vi "Model - Init.vi"(8 "error in (no error)":errorcluster) -> (0 "error out":errorcluster, 3 "View Model":T1)   [LabVIEW 2017]
doc: "Initialize all View Model Components."
uses:
  Controls/View Model.ctl
  Controls/Shared Model.ctl
  Error Handler/Controls/Error Model.ctl
  Error Handler/Controls/Error Data.ctl
  Error Handler/Controls/Error Type.ctl
  Error Handler/Controls/Error Source.ctl
  Configuration/Controls/Config Model.ctl
  Configuration/Controls/Config CMD.ctl
  Configuration/Controls/Config Command.ctl
  Controller/Controls/Controller Model.ctl
  Controller/Controls/Controller Overhead.ctl
  Controller/Controls/Controller Transaction.ctl
  Controller/Controls/Controller State.ctl
  Configuration/Controls/Config Data Record.ctl
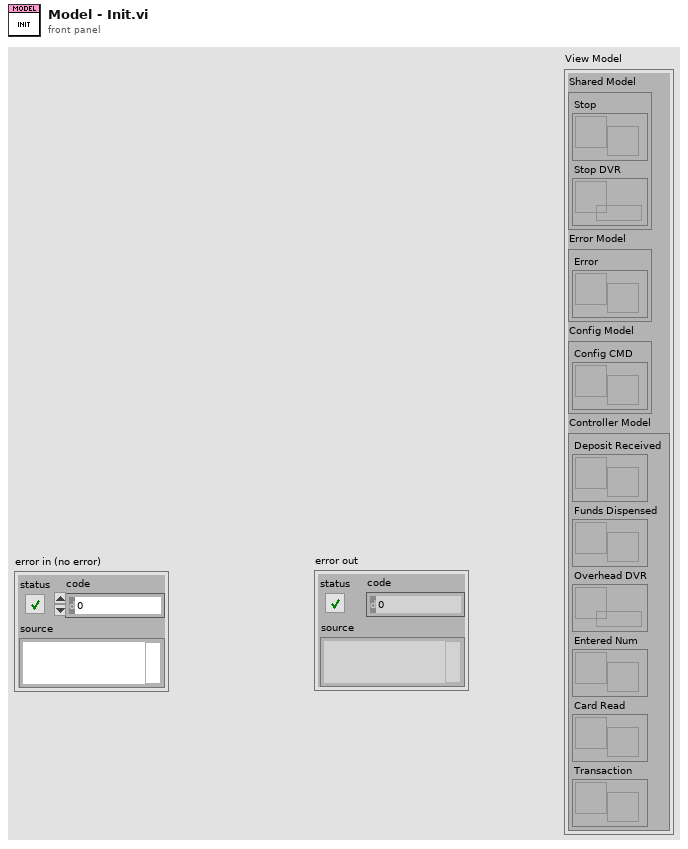
[diagram p1: front panel]
types:
  T1 = typedef "View Model.ctl" = cluster{"Shared Model":T2, "Error Model":T3, "Config Model":T4, "Controller Model":T5}
  T2 = typedef "Shared Model.ctl" = cluster{"Stop":refnum<user-event>, "Stop DVR":refnum<data-value>}
  T3 = typedef "Error Model.ctl" = cluster{"Error":refnum<user-event>}
  T4 = typedef "Config Model.ctl" = cluster{"Config CMD":refnum<user-event>}
  T5 = typedef "Controller Model.ctl" = cluster{"Deposit Received":refnum<user-event>, "Funds Dispensed":refnum<user-event>, "Overhead DVR":refnum<data-value>, "Entered Num":refnum<user-event>, "Card Read":refnum<user-event>, "Transaction":refnum<user-event>}
  T6 = typedef "Controller Transaction.ctl" = enum16{"Balance Inquiry", "Deposit", "Withdrawal", "Fast Cash", "New Transaction", "Terminate Session"}
  T7 = typedef "Controller Overhead.ctl" = cluster{"Account Number":u32, "Amount":u32, "Transaction":T6, "Current State":T8, "Next State":T8, "Elapsed Time":dbl, "User Messages":string[], "Data Record":T9, "Account Found?":bool, "Invalid Login":u8, "Message":string}
  T8 = typedef "Controller State.ctl" = enum16{"Idle", "Initial", "Login", "Balance Inquiry", "Deposit", "Withdrawal", "Fast Cash", "Terminate"}
  T9 = typedef "Config Data Record.ctl" = cluster{"Account Number":u32, "First Name":string, "Last Name":string, "Balance":dbl}
  T10 = typedef "Config CMD.ctl" = cluster{"CMD":T11, "Data":variant}
  T11 = typedef "Config Command.ctl" = enum16{"Read", "Search", "Update"}
  T12 = typedef "Error Data.ctl" = cluster{"Error Type":T13, "Error Source":T14, "Data":variant}
  T13 = typedef "Error Type.ctl" = enum16{"Console Error", "Sensor Interface IO Error", "Process Step Error"}
  T14 = typedef "Error Source.ctl" = enum16{"User Console", "Display Console", "Sensor Interface"}
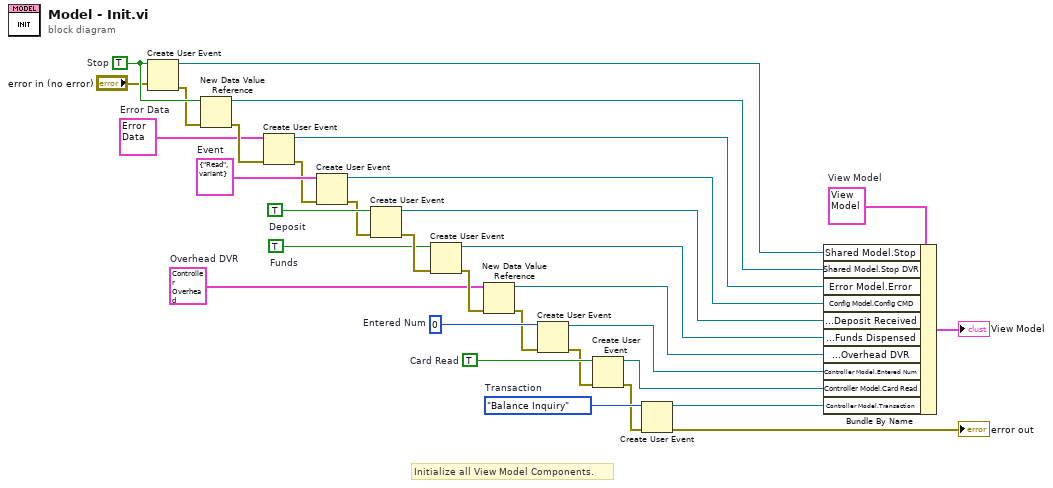
[diagram p0: block diagram]
diagram:
  w14 = Controller_Transaction."Balance Inquiry"  # Transaction
  w16 = TRUE  # Card Read
  w18 = 0  # Entered Num
  w1 = T7 {"Account Number"=0, "Amount"=0, "Transaction"=enum."Balance Inquiry", "Current State"=enum."Balance Inquiry", "Next State"=enum."Idle", "Elapsed Time"=0.0, "User Messages"=[], "Data Record"={"Account Number"=0, "First Name"="", "Last Name"="", "Balance"=0.0}, "Account Found?"=FALSE, "Invalid Login"=0, "Message"=""}  # Overhead DVR
  w20 = TRUE  # Funds
  w23 = TRUE  # Deposit
  w25 = T10 {"CMD"=enum."Read", "Data"=variant}  # Event
  w26 = T12 {"Error Type"=enum."Console Error", "Error Source"=enum."User Console", "Data"=variant}  # Error Data
  w30 = TRUE  # Stop
  w32 = T1 {"Shared Model"={"Stop"=refnum, "Stop DVR"=refnum}, "Error Model"={"Error"=refnum}, "Config Model"={"Config CMD"=refnum}, "Controller Model"={"Deposit Received"=refnum, "Funds Dispensed"=refnum, "Overhead DVR"=refnum, "Entered Num"=refnum, "Card Read"=refnum, "Transaction"=refnum}}  # View Model
  # "Initialize all View Model Components."
  n1 = Create User Event(user event datatype=w30, error in="error in (no error)") -> (user event=w2:refnum<user-event>, error out=w29:errorcluster)
  n2 = New Data Value Reference(data value=w30, error in=w29) -> (data value reference=w3:refnum<data-value>, error out=w27:errorcluster)
  n3 = Create User Event(user event datatype=w26, error in=w27) -> (user event=w4:refnum<user-event>, error out=w24:errorcluster)
  n4 = Create User Event(user event datatype=w25, error in=w24) -> (user event=w5:refnum<user-event>, error out=w22:errorcluster)
  n5 = Create User Event(user event datatype=w23, error in=w22) -> (user event=w6:refnum<user-event>, error out=w21:errorcluster)
  n6 = Create User Event(user event datatype=w20, error in=w21) -> (user event=w7:refnum<user-event>, error out=w19:errorcluster)
  n7 = New Data Value Reference(data value=w1, error in=w19) -> (data value reference=w8:refnum<data-value>, error out=w17:errorcluster)
  n8 = Create User Event(user event datatype=w18, error in=w17) -> (user event=w9:refnum<user-event>, error out=w15:errorcluster)
  n9 = Create User Event(user event datatype=w16, error in=w15) -> (user event=w10:refnum<user-event>, error out=w13:errorcluster)
  n10 = Create User Event(user event datatype=w14, error in=w13) -> (user event=w12:refnum<user-event>, error out=→"error out":errorcluster)
  n11 = Bundle By Name(cluster=w32, "Shared Model.Stop"=w2, "Shared Model.Stop DVR"=w3, "Error Model.Error"=w4, "Config Model.Config CMD"=w5, "Controller Model.Deposit Received"=w6, "Controller Model.Funds Dispensed"=w7, "Controller Model.Overhead DVR"=w8, "Controller Model.Entered Num"=w9, "Controller Model.Card Read"=w10, "Controller Model.Transaction"=w12) -> (→"View Model":T1)
